vi "Get PC name.vi"(8 "error in (no error)":errorcluster) -> (0 "error out":errorcluster, 3 "Hostname":string)   [LabVIEW 2026, in "TALOS.lvlib"]
doc: "This VI gets the PC name, and convert it to lowcase letters (to avoid name conflict with other services, like SV)."
uses:
  TALOS.lvlib
  Global Memory.vi
  <resource>/objmgr/nisysapi.rc
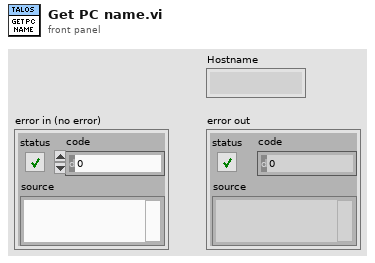
[diagram p1: front panel]
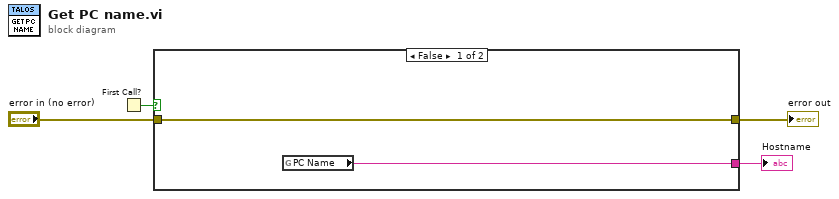
[diagram p0: block diagram]
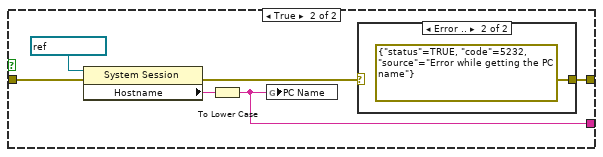
[diagram p2: hidden frame]
diagram:
  n1 = First Call?() -> (First Call?: T/F=w1:bool)
  n2 = case shown="False" w1 {
    tunnel: [w6 w7] -> w4
    tunnel: "error in (no error)" -> [w6 w12]
    tunnel: [w5 w9] -> w2
    frame False {
      n3 = global read "Global Memory.vi" "PC Name"() -> (w5:string)
    }
    frame True {
      n4 = property class="System Session"(reference=refnum<k21> "localhost" ("System Session"), error in=w12) -> (error out=w8:errorcluster, "Hostname"=w10:string)  [unwired: 1 out]
      n5 = To Lower Case(string=w10) -> (all lower case string=w9:string)
      n6 = global write "Global Memory.vi" "PC Name"(w9) -> ()
      n7 = case shown="Error .." w8 {
        selector: w8 -> [w13 _]
        tunnel: [w13 errorcluster {"status"=TRUE, "code"=5232, "source"="Error while getting the PC name"} ("error IO")] -> w7
        frame No Error {
        }
        frame Error {
        }
      }
    }
  }
  "error out" <- w4
  "Hostname" <- w2
